vi "CommonDialogSingleBttn.vi"() -> (2 "Message":string, 3 "Cancelled?":bool)   [LabVIEW 2021]
doc: "Use this template to create a dialog box with event handling."
uses:
  <vilib>/Platform/browser.llb/Open URL in Default Browser (string).vi
panel:
  in  "DatabaseSetup":bool
  in  "Hyperlinkpath":bool
  in  "OK":bool
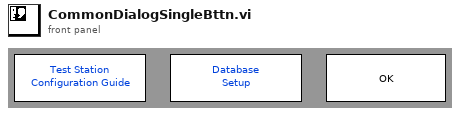
[diagram p1: front panel]
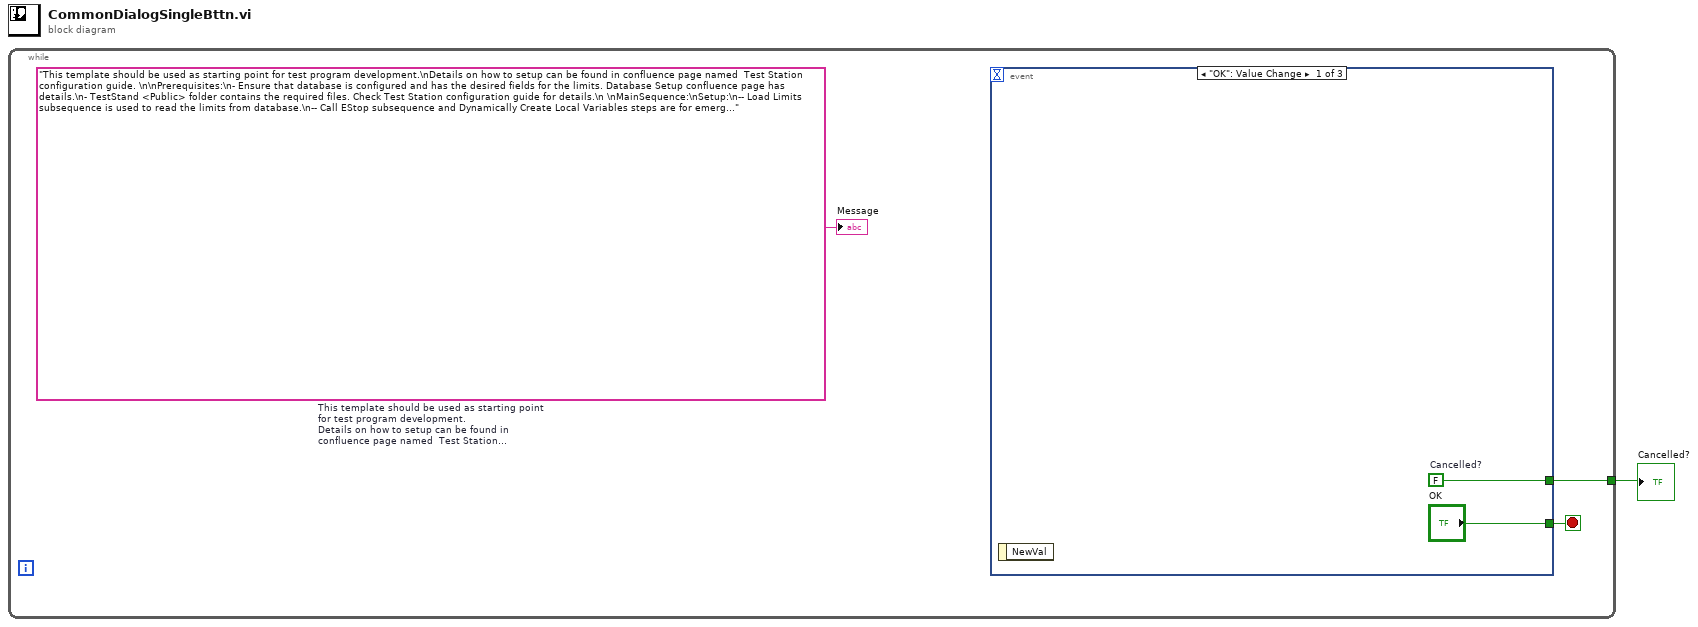
[diagram p0: block diagram]
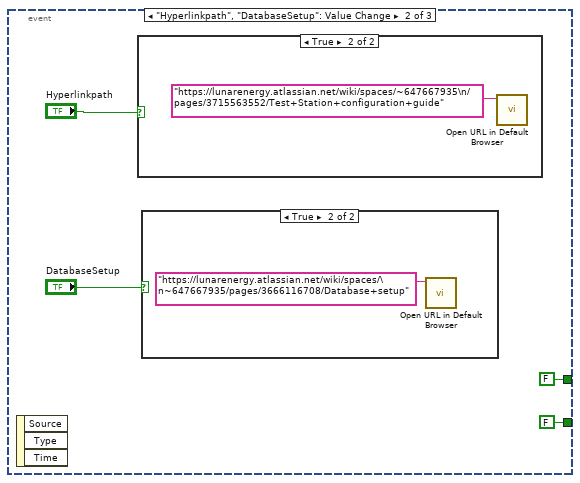
[diagram p2: hidden frame]
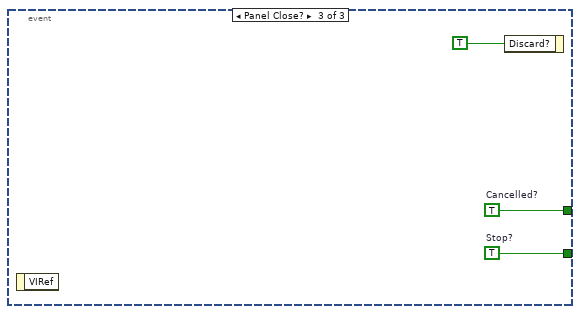
[diagram p5: hidden frame]
diagram:
  n1 = while {
    tunnel: [w3] -> w1
    stop <- w4 stop-if-true
    w2 = "This template should be used as starting point for test program development.\nDetails on how to setup can be found in confluence page named  Test Station configuration guide. \n\nPrerequisites:\n- Ensure that database is configured and has the desired fields for the limits. Database Setup confluence page has details.\n- TestStand <Public> folder contains the required files. Check Test Station configuration guide for details.\n \nMainSequence:\nSetup:\n-- Load Limits subsequence is used to read the limits from database.\n-- Call EStop subsequence and Dynamically Create Local Variables steps are for emergency stop functionality.\n\nMain:\n-- Implement DUT specific functions in this section. Template only provides examples of using different step types and custom waveform step types.\n\nCleanup:\n-- Kill EStop Execution step is part of emergency stop.\n\nCopy the template sequence in the DUT specific folder and rename it to DUT specific name.\nDelete SequenceFileLoad callback  from DUT specific sequence file\n\nNote: To dry-run template with lunardb sample database use the Barcode as: P:10-000001R:0AS:ABC220212345 "  # This template should be used as starting point for test program development. Details on how to setup can be found in confluence page named  Test Station configuration guide.   Prerequisites: - Ensure that database is configured and has the desired fields for the limits. Database Setup confluence page has details. - TestStand <Public> folder contains the required files. Check Test Station configuration guide for details.   MainSequence: Setup: -- Load Limits subsequence is used to read the limits from database. -- Call EStop subsequence and Dynamically Create Local Variables steps are for emergency stop functionality.  Main: -- Implement DUT specific functions in this section. Template only provides examples of using different step types and custom waveform step types.  Cleanup: -- Kill EStop Execution step is part of emergency stop.  Copy the template sequence in the DUT specific folder and rename it to DUT specific name. Delete SequenceFileLoad callback  from DUT specific sequence file  Note: To dry-run template with lunardb sample database use the Barcode as: P:10-000001R:0AS:ABC220212345
    n2 = event shown="[0] \"OK\": Value Change" {
      selector: _ -> [_ _ _]
      dyn-events: _ -> [_ _ _]
      timeout: _ -> [_ _ _]
      tunnel: ["OK" FALSE ("Stop?") w14] -> w4
      tunnel: [w6 FALSE ("Cancelled?") w13] -> w3
      event "OK": Value Change {
        w6 = FALSE  # Cancelled?
        n3 = event-data() -> ()  [unwired: 1 in, 1 out]
      }
      event "Hyperlinkpath", "DatabaseSetup": Value Change {
        n4 = event-data() -> ()  [unwired: 1 in, 3 out]
        n5 = case shown="True" "Hyperlinkpath" {
          frame False {
          }
          frame True {
            n6 = call-poly <vilib>:"Open URL in Default Browser.vi"("URL"="https://lunarenergy.atlassian.net/wiki/spaces/~647667935\n/pages/3715563552/Test+Station+configuration+guide") -> ()  [unwired: 5 in, 2 out]
          }
        }
        n7 = case shown="True" "DatabaseSetup" {
          frame False {
          }
          frame True {
            n8 = call-poly <vilib>:"Open URL in Default Browser.vi"("URL"="https://lunarenergy.atlassian.net/wiki/spaces/\n~647667935/pages/3666116708/Database+setup") -> ()  [unwired: 5 in, 2 out]
          }
        }
      }
      event Panel Close? {
        w13 = TRUE  # Cancelled?
        w14 = TRUE  # Stop?
        n9 = event-data() -> ()  [unwired: 1 in, 1 out]
        n10 = event-data("Discard?"=TRUE) -> ()  [unwired: 1 in, 1 out]
      }
    }
    "Message" <- w2
  }
  "Cancelled?" <- w1
